vi "PutStr16.vi"(8 "error in (no error)":errorcluster, 9 "Size":i32, 10 "string":string, 11 "MsgPackSerializer in":refnum<class "MsgPackSerializer.lvclass">) -> (0 "error out":errorcluster, 3 "MsgPackSerializer out":refnum<class "MsgPackSerializer.lvclass">)   [LabVIEW 2015, in "MsgPackSerializer.lvclass"]
uses:
  MsgPackSerializer.lvclass
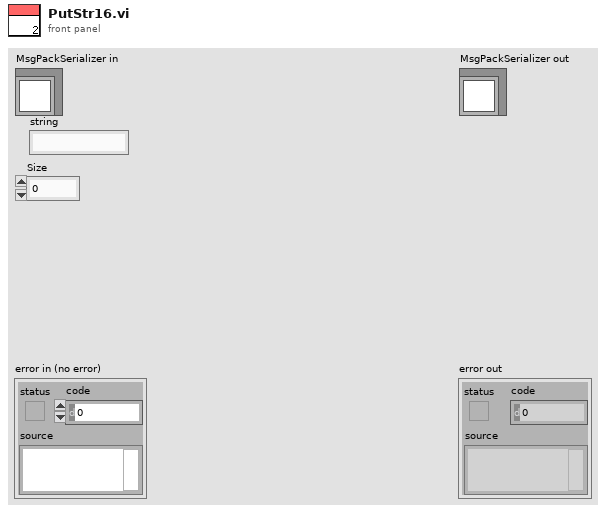
[diagram p1: front panel]
types:
  T1 = enum16{"big-endian, network order", "native, host order", "little-endian"}
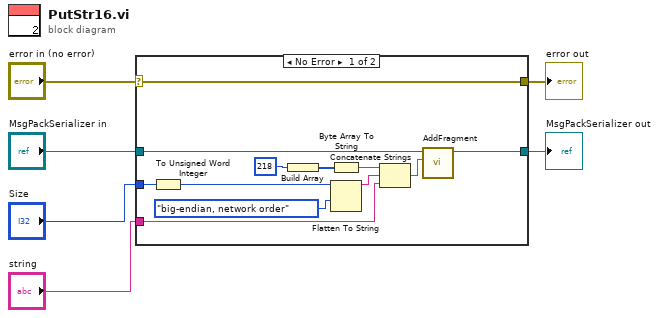
[diagram p0: block diagram]
diagram:
  n1 = case shown="No Error" "error in (no error)" {
    selector: "error in (no error)" -> [w18 w20]
    tunnel: [w18 w20] -> w5
    tunnel: [w16 w19] -> w3
    tunnel: "MsgPackSerializer in" -> [w17 w19]
    tunnel: "string" -> [w8 _]
    tunnel: "Size" -> [w7 _]
    frame No Error {
      n2 = To Unsigned Word Integer(number=w7) -> (unsigned 16bit integer=w15:u16)
      n3 = Build Array(u8 218 ("Number")) -> (w12:u8[])
      n4 = Byte Array To String(unsigned byte array=w12) -> (string=w10:string)
      n5 = Flatten To String(anything=w15, byte order (0:big-endian, network order)=T1."big-endian, network order") -> (data string=w9:string)  [unwired: 2 in, 2 out]
      n6 = Concatenate Strings(w10, w9, w8) -> (w13:string)
      n7 = call "AddFragment.vi"("Fragment"=w13, "MsgPackSerializer in"=w17) -> ("MsgPackSerializer out"=w16:refnum<class "MsgPackSerializer.lvclass">)  [unwired: 8 in, 1 out]
    }
    frame Error {
    }
  }
  "error out" <- w5
  "MsgPackSerializer out" <- w3
